vi "Get Basic Audio File Info - Copy.vi"(8 "error in (no error)":errorcluster, 11 "Audio File Refnum In":refnum<file>) -> (0 "error out":errorcluster, 1 "sample_rate":u32, 2 "channels":u32, 3 "Audio File Refnum Out":refnum<file>, 4 "read_offset":u64)   [LabVIEW 2020]
doc: "Get basic audio information about the file."
uses:
  <vilib>/Utility/error.llb/Error Cluster From Error Code.vi
  <vilib>/Dataflow_G/G-Audio/G-Audio.lvlib
  github/dataflowg/g-audio/src/.LabVIEW/G-Audio/lib/g_audio_x64.dll
  <vilib>/Dataflow_G/G-Audio/lib/g_audio_x86.dll
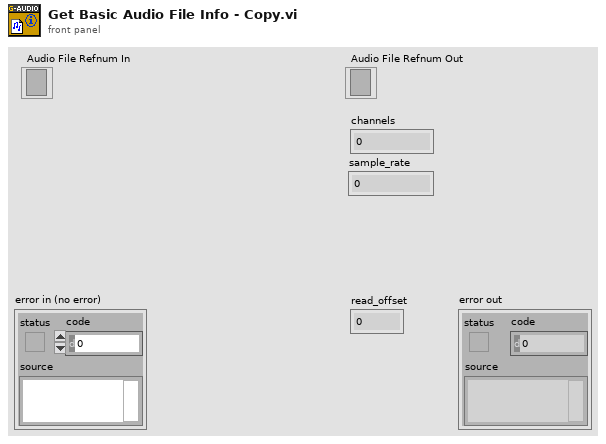
[diagram p1: front panel]
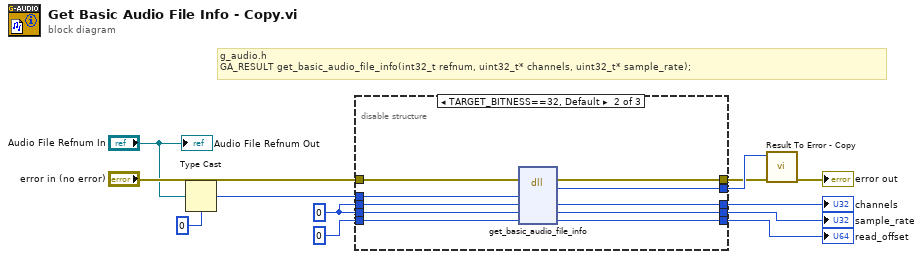
[diagram p0: block diagram]
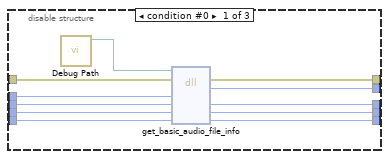
[diagram p2: hidden frame]
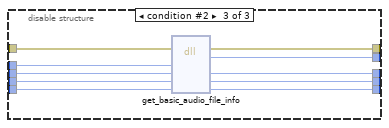
[diagram p3: hidden frame]
diagram:
  w8 = u32 0
  # "g_audio.h\nGA_RESULT get_basic_audio_file_info(int32_t refnum, uint32_t* channels, uint32_t* sample_rate);"
  n1 = Type Cast(type=0, x="Audio File Refnum In") -> (*(type *) &x=w9:i32)
  n2 = disable-structure shown="TARGET_BITNESS==32, Default" {
    disable-tunnel: "error in (no error)" -> [w23 w33 w43]
    disable-tunnel: [w16 w26 w36] -> w5
    disable-tunnel: [w22 w32 w42] -> w4
    disable-tunnel: [w17 w27 w37] -> w6
    disable-tunnel: w9 -> [w21 w31 w41]
    disable-tunnel: w8 -> [w20 w30 w40]
    disable-tunnel: w8 -> [w19 w29 w39]
    disable-tunnel: [w18 w28 w38] -> w7
    disable-tunnel: u64 0 -> [w14 w25 w35]
    disable-tunnel: [w13 w24 w34] -> w1
    frame condition #0 {
      n3 = call <vilib>:"Debug Path.vi"() -> ("Debug Path"=w15:path)  [unwired: 11 in]
      n4 = dll-call lib="?" fn="get_basic_audio_file_info"(path in=w15, error in=w23, "refnum"=w21, "channels"=w20, "sample_rate"=w19, "read_offset"=w14) -> (error out=w22:errorcluster, "result"=w16:i32, "channels"=w18:u32, "sample_rate"=w17:u32, "read_offset"=w13:u64)  [unwired: 2 in, 1 out]
    }
    frame condition #1 (active) {
      n5 = dll-call lib="C:/Program Files (x86)/National Instruments/LabVIEW 2020/vi.lib/Dataflow_G/G-Audio/lib/g_audio_x86.*" fn="get_basic_audio_file_info"(error in=w33, "refnum"=w31, "channels"=w30, "sample_rate"=w29, "read_offset"=w25) -> (error out=w32:errorcluster, "result"=w26:i32, "channels"=w28:u32, "sample_rate"=w27:u32, "read_offset"=w24:u64)  [unwired: 3 in, 1 out]
    }
    frame condition #2 {
      n6 = dll-call lib="C:/github/dataflowg/g-audio/src/LabVIEW/G-Audio/lib/g_audio_x64.*" fn="get_basic_audio_file_info"(error in=w43, "refnum"=w41, "channels"=w40, "sample_rate"=w39, "read_offset"=w35) -> (error out=w42:errorcluster, "result"=w36:i32, "channels"=w38:u32, "sample_rate"=w37:u32, "read_offset"=w34:u64)  [unwired: 3 in, 1 out]
    }
  }
  "channels" <- w7
  "sample_rate" <- w6
  "read_offset" <- w1
  n7 = call "Result To Error - Copy.vi"("error in (no error)"=w4, "Result Code"=w5) -> ("error out"=→"error out":errorcluster)  [unwired: 9 in]
  "Audio File Refnum Out" <- "Audio File Refnum In"
